vi "WAPIAerReadPosition.vi"(3 "nAxis":i16(ring) items=["Axis 1", "Axis 2", "Axis 3", "Axis 4"], 7 "nType":i16(ring) items=["Relative, commanded, not real time", "Absolute, commanded, not real time", "Real time, feedback", "Real time, commanded"], 9 "error in (no error)":errorcluster) -> (0 "Position":dbl, 6 "error out":errorcluster)   [LabVIEW 2009]
uses:
  win50032.dll
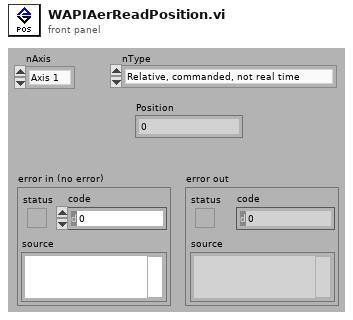
[diagram p1: front panel]
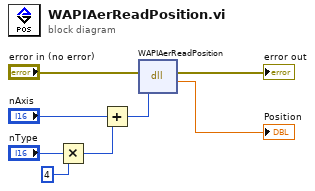
[diagram p0: block diagram]
diagram:
  n1 = Multiply(x="nType", y=i16 4) -> (x*y=w3:i16)
  n2 = Add(x="nAxis", y=w3) -> (x+y=w5:i16)
  n3 = dll-call lib="win50032.dll" fn="WAPIAerReadPosition"(error in="error in (no error)", "nPos"=w5) -> (error out=→"error out":errorcluster, "return type"=→"Position":dbl)  [unwired: 3 in, 1 out]
